vi "Shift_Register.vi"() -> ()   [LabVIEW 2019]
panel:
  out "Previo Intr":u16
  out "Current Intr":u16
  in  "stop":bool
  out "Result":u16
  in  "Numeric":u16
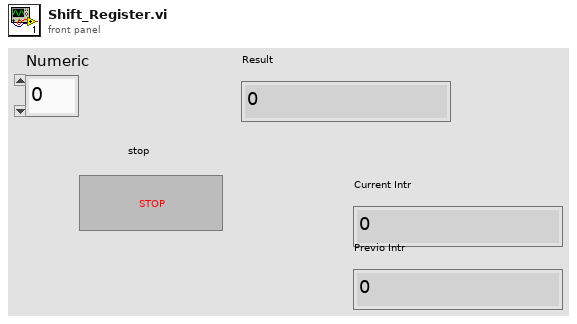
[diagram p1: front panel]
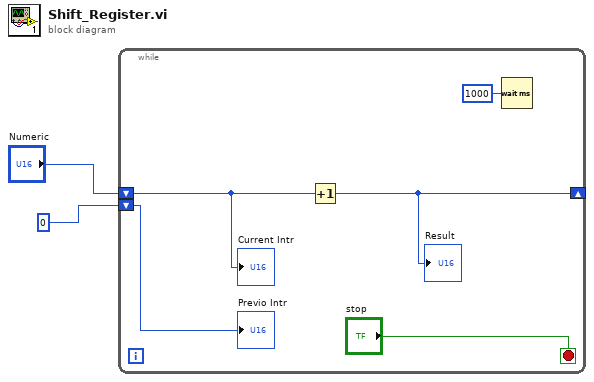
[diagram p0: block diagram]
diagram:
  n1 = while {
    shift-right: [w7] -> _
    shift-left: "Numeric" -> [w4]
    shift-left: u16 0 ("Numeric") -> [w3]
    stop <- "stop" stop-if-true
    n2 = Increment(x=w4) -> (x+1=w7:u16)
    "Result" <- w7
    n3 = Wait (ms)(milliseconds to wait=u32 1000) -> ()  [unwired: 1 out]
    "Current Intr" <- w4
    "Previo Intr" <- w3
  }
